vi "RescalingDomain_subvi.vi"(8 "min":dbl, 9 "max":dbl, 10 "numbins":dbl, 11 "Domain":dbl[][](array[numeric])) -> (3 "RescaledDomain":dbl[][](array[numeric]))   [LabVIEW 2019]
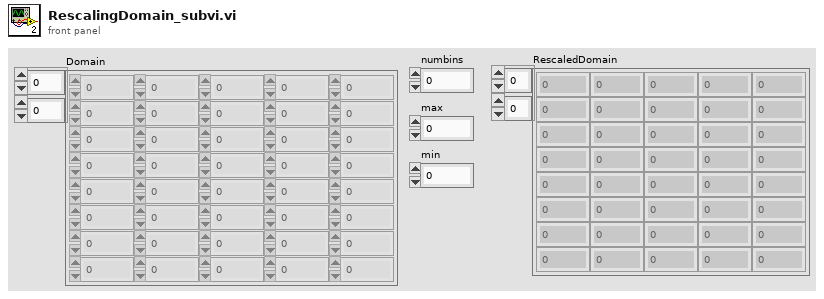
[diagram p1: front panel]
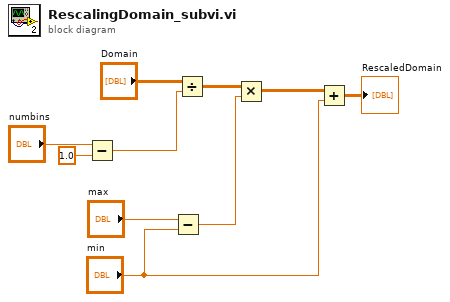
[diagram p0: block diagram]
diagram:
  n1 = Subtract(x="numbins", y=1.0) -> (x-y=w6:dbl)
  n2 = Subtract(x="max", y="min") -> (x-y=w9:dbl)
  n3 = Divide(x="Domain", y=w6) -> (x/y=w10:dbl[][])
  n4 = Multiply(x=w10, y=w9) -> (x*y=w3:dbl[][])
  n5 = Add(x=w3, y="min") -> (x+y=→"RescaledDomain":dbl[][])
